vi "Test MultiValue INSERT.vi"(9 "file (use dialog)":path, 10 "Method":T1(ring), 11 "Numeric":i32=1000000) -> (2 "Rows/sec":dbl format="%#_3p", 3 "Time per row":dbl format="%#_3p")   [LabVIEW 2019]
uses:
  <vilib>/JDP Science/PostgreSQL Library/Connection/Execute Command (No results).vi
  <vilib>/JDP Science/PostgreSQL Library/Connection/Execute (no results).vi
  <vilib>/JDP Science/PostgreSQL Library/Connection/Execute (Return first result with rows).vi
  <vilib>/JDP Science/PostgreSQL Library/Connection/Execute Command (Result).vi
  <vilib>/JDP Science/PostgreSQL Library/Result/Clear.vi
  <vilib>/JDP Science/PostgreSQL Library/Connection/Execute Single Statement (String Parameters).vi
  <userlib>/_OpenG.lib/string/string.llb/Trim Whitespace (String)__ogtk.vi
  <vilib>/JDP Science/PostgreSQL Library/Connection/PQ Connection.lvclass
panel:
  out "concatenated string":string
  in  "Connection Strings to access PostgreSQL":string="host=localhost port=5432 dbname = mydb "
  out "error out":errorcluster
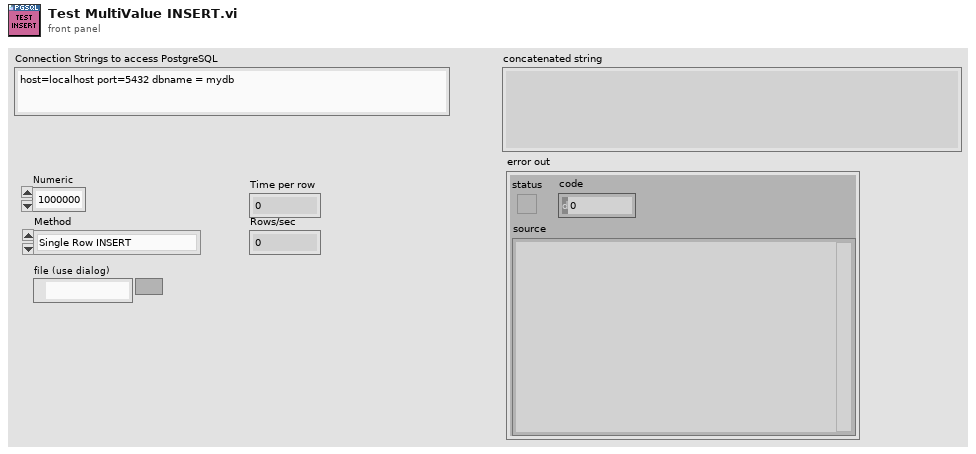
[diagram p1: front panel]
types:
  T1 = enum16{"Single Row INSERT", "Multi Row INSERT", "COPY", "COPY file"}
  T2 = typedef "PQ Result.lvclass/Parameter Type.ctl" = enum16{"Text", "ByteA", "Integer", "SGL", "DBL", "Timestamp", "Enum", "Boolean", "Array", "NULL", "Unsupported"}
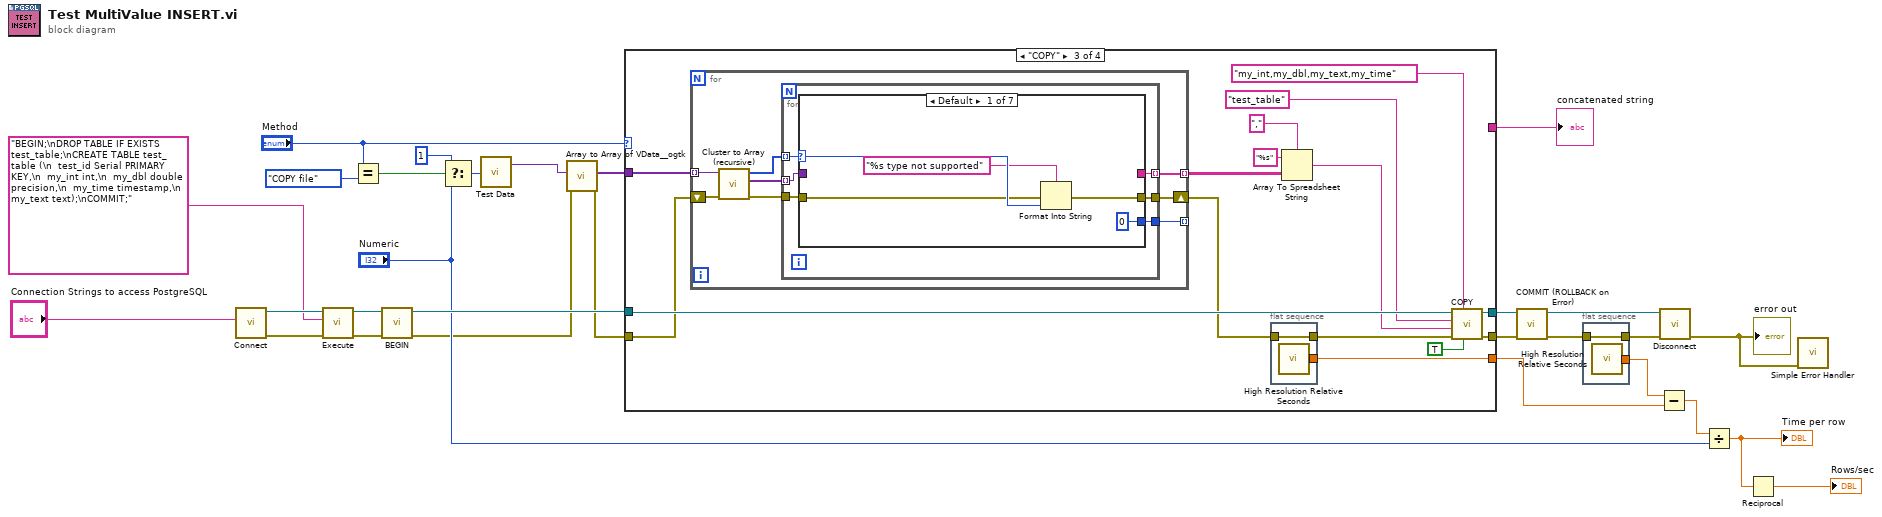
[diagram p0: block diagram]
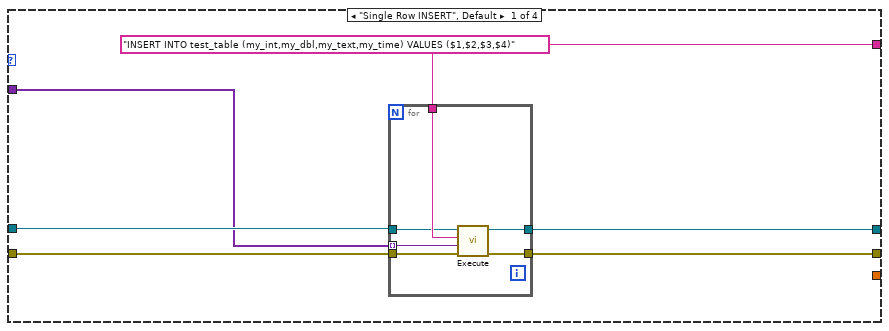
[diagram p2: hidden frame]
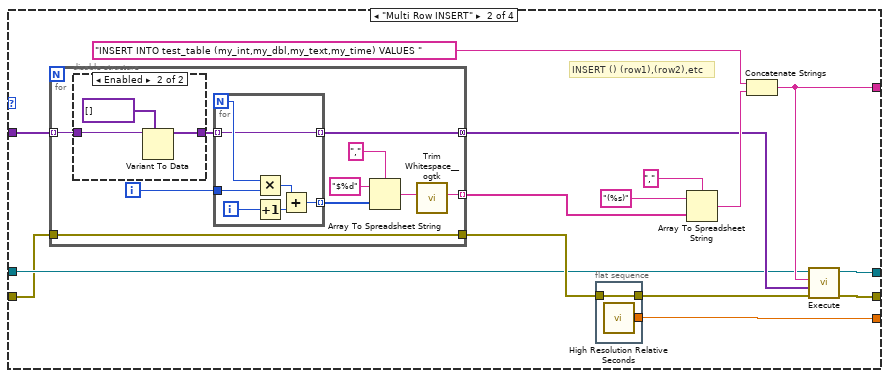
[diagram p3: hidden frame]
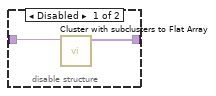
[diagram p4: hidden frame]
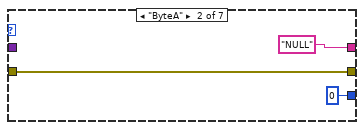
[diagram p5: hidden frame]
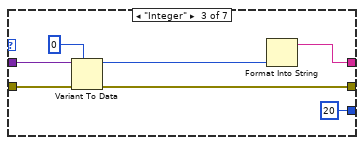
[diagram p6: hidden frame]
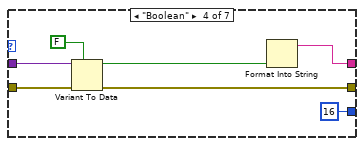
[diagram p7: hidden frame]
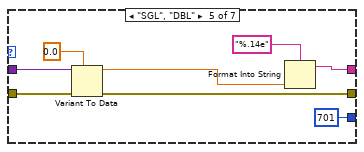
[diagram p8: hidden frame]
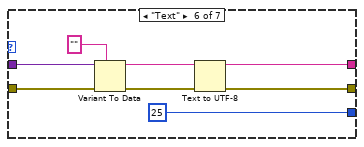
[diagram p9: hidden frame]
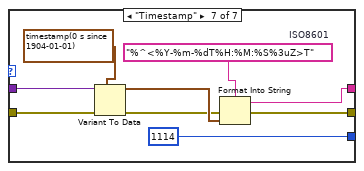
[diagram p10: hidden frame]
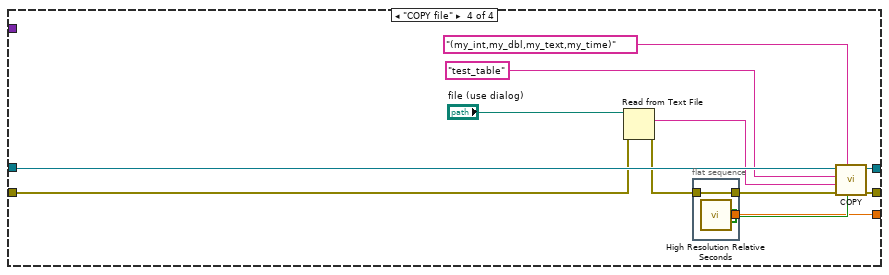
[diagram p11: hidden frame]
diagram:
  n1 = call <vilib>:"Connect.vi"("Connection Strings"="Connection Strings to access PostgreSQL") -> ("error out"=w25:errorcluster, "PQ Connection"=w27:refnum<class "PQ Connection.lvclass">)  [unwired: 9 in]
  n2 = call-poly <vilib>:"Execute.vi"("error in (no error)"=w25, "SQL"="BEGIN;\nDROP TABLE IF EXISTS test_table;\nCREATE TABLE test_table (\n  test_id Serial PRIMARY KEY,\n  my_int int,\n  my_dbl double precision,\n  my_time timestamp,\n  my_text text);\nCOMMIT;", "PQ Connection in"=w27) -> ("error out"=w13:errorcluster, "PQ Connection out"=w26:refnum<class "PQ Connection.lvclass">)  [unwired: 7 in]
  n3 = Equal?(x="Method", y=T1."COPY file") -> (x = y?=w9:bool)
  n4 = call <vilib>:"BEGIN.vi"("error in (no error)"=w13, "PQ Connection in"=w26) -> ("error out"=w2:errorcluster, "PQ Connection out"=w6:refnum<class "PQ Connection.lvclass">)  [unwired: 8 in]
  n5 = Select(t=1, s=w9, f="Numeric") -> (s? t:f=w8:i32)
  n6 = call "Test Data.vi"("Size"=w8) -> ("Data"=w14:variant)  [unwired: 1 out]
  n7 = call <userlib>:"Array to Array of VData__ogtk.vi"("error in (no error)"=w2, "MultiD Array"=w14) -> ("error out"=w1:errorcluster, "1D Array of Variants"=w3:variant[])  [unwired: 8 in]
  n8 = case shown="\"COPY\"" "Method" {
    tunnel: w3 -> [w31 w44 w83 _]
    tunnel: w6 -> [w34 w45 w95 w170]
    tunnel: [w32 w52 w93 w168] -> w17
    tunnel: [w33 w51 w94 w169] -> w16
    tunnel: w1 -> [w35 w43 w82 w160]
    tunnel: [w30 w50 _ _] -> w15
    tunnel: [_ w46 w84 w161] -> w7
    frame "Single Row INSERT", Default {
      w30 = "INSERT INTO test_table (my_int,my_dbl,my_text,my_time) VALUES ($1,$2,$3,$4)" ("command")
      n9 = for {
        tunnel: w30 -> [w40]
        tunnel: w31 -> [w36] mode=indexing
        tunnel: w34 -> [w39]
        tunnel: [w41] -> w32
        tunnel: w35 -> [w38]
        tunnel: [w37] -> w33
        n10 = call-poly <vilib>:"Execute.vi"("error in (no error)"=w38, "Parameters"=w36, "SQL"=w40, "PQ Connection in"=w39) -> ("error out"=w37:errorcluster, "PQ Connection out"=w41:refnum<class "PQ Connection.lvclass">)  [unwired: 6 in]
      }
    }
    frame "Multi Row INSERT" {
      # "INSERT () (row1),(row2),etc"
      n11 = for {
        tunnel: w44 -> [w68] mode=indexing
        tunnel: [w60] -> w42 mode=indexing
        tunnel: [w61] -> w49 mode=concatenating
        tunnel: w43 -> [w59]
        tunnel: [w59] -> w48
        i -> [w66]
        n12 = disable-structure shown="Enabled" {
          disable-tunnel: w68 -> [w70 w72]
          disable-tunnel: [w69 w71] -> w67
          frame Disabled {
            n13 = call <vilib>:"Cluster with subclusters to Flat Array.vi"("Variant"=w70) -> ("Array of items"=w69:variant[])  [unwired: 8 in, 2 out]
          }
          frame Enabled {
            n14 = Variant To Data(type=variant[] [], Variant=w72) -> (data=w71:variant[])  [unwired: 1 in, 1 out]
          }
        }
        n15 = for {
          N -> [w79]
          tunnel: w67 -> [w75] mode=indexing
          tunnel: w66 -> [w78]
          tunnel: [w76] -> w65 mode=indexing
          tunnel: [w75] -> w61 mode=indexing
          i -> [w80]
          n16 = Multiply(x=w79, y=w78) -> (x*y=w77:i32)
          n17 = Increment(x=w80) -> (x+1=w74:i32)
          n18 = Add(x=w77, y=w74) -> (x+y=w76:i32)
        }
        n19 = Array To Spreadsheet String(delimiter (Tab)=",", array=w65, 3:"$%d" ("format string")) -> (spreadsheet string=w62:string)
        n20 = call-poly <userlib>:"Trim Whitespace__ogtk.vi"("String in"=w62) -> ("String out"=w60:string)  [unwired: 6 in]
      }
      n21 = flat-sequence {
        tunnel: w48 -> [w58]
        tunnel: [w58] -> w47
        tunnel: [w57] -> w46
        frame #0 {
          n22 = call <vilib>:"High Resolution Relative Seconds.vi"() -> ("relative seconds"=w57:dbl)
        }
      }
      n23 = Array To Spreadsheet String(delimiter (Tab)=",", array=w42, 3:"(%s)" ("format string")) -> (spreadsheet string=w53:string)
      n24 = Concatenate Strings("INSERT INTO test_table (my_int,my_dbl,my_text,my_time) VALUES " ("command"), w53) -> (w50:string)
      n25 = call-poly <vilib>:"Execute.vi"("error in (no error)"=w47, "Parameters"=w49, "SQL"=w50, "PQ Connection in"=w45) -> ("error out"=w51:errorcluster, "PQ Connection out"=w52:refnum<class "PQ Connection.lvclass">)  [unwired: 6 in]
    }
    frame "COPY" {
      n26 = for {
        tunnel: [w105] -> w91 mode=indexing
        shift-right: [w104] -> w81
        shift-left: w82 -> [w102]
        tunnel: [w103] -> _ mode=indexing
        tunnel: w83 -> [w101] mode=indexing
        n27 = call <vilib>:"Cluster to Array (recursive).vi"("error in (no error)"=w102, "Variant"=w101) -> ("error out"=w98:errorcluster, "Elements"=w100:variant[], "Types"=w99:T2[])  [unwired: 6 in, 1 out]
        n28 = for {
          tunnel: [w111] -> w105 mode=indexing
          tunnel: [w110] -> w104
          tunnel: [w109] -> w103
          tunnel: w100 -> [w107] mode=indexing
          tunnel: w99 -> [w108] mode=indexing
          tunnel: w98 -> [w106]
          n29 = case shown="Default" w108 {
            selector: w108 -> [w116 _ _ _ _ _ _]
            tunnel: w107 -> [_ _ w126 w133 w141 w149 w158]
            tunnel: [_ "NULL" w123 w131 w138 w144 w150] -> w111
            tunnel: w106 -> [w114 w118 w122 w130 w136 w147 w157]
            tunnel: [w113 w118 w121 w129 w135 w142 w151] -> w110
            tunnel: [0 0 20 16 701 25 1114] -> w109
            frame Default {
              n30 = Format Into String(format string="%s type not supported", error in=w114, w116) -> (error out=w113:errorcluster)  [unwired: 1 in, 1 out]
            }
            frame "ByteA" {
            }
            frame "Integer" {
              n31 = Variant To Data(error in=w122, type=i64 0, Variant=w126) -> (data=w124:i64, error out=w121:errorcluster)
              n32 = Format Into String(w124) -> (resulting string=w123:string)  [unwired: 3 in, 1 out]
            }
            frame "Boolean" {
              n33 = Variant To Data(error in=w130, type=FALSE, Variant=w133) -> (data=w132:bool, error out=w129:errorcluster)
              n34 = Format Into String(w132) -> (resulting string=w131:string)  [unwired: 3 in, 1 out]
            }
            frame "SGL", "DBL" {
              n35 = Variant To Data(error in=w136, type=0.0, Variant=w141) -> (data=w139:dbl, error out=w135:errorcluster)
              n36 = Format Into String(format string="%.14e", w139) -> (resulting string=w138:string)  [unwired: 2 in, 1 out]
            }
            frame "Text" {
              n37 = Variant To Data(error in=w147, type="", Variant=w149) -> (data=w145:string, error out=w143:errorcluster)
              n38 = Text to UTF-8(8:w143, 11:w145) -> (0:w142:errorcluster, 3:w144:string)  [unwired: 1 in]
            }
            frame "Timestamp" {
              w154 = "%^<%Y-%m-%dT%H:%M:%S%3uZ>T"  # ISO8601
              n39 = Variant To Data(error in=w157, type=timestamp(0 s since 1904-01-01), Variant=w158) -> (data=w153:timestamp, error out=w152:errorcluster)
              n40 = Format Into String(format string=w154, error in=w152, w153) -> (resulting string=w150:string, error out=w151:errorcluster)  [unwired: 1 in]
            }
          }
        }
      }
      n41 = flat-sequence {
        tunnel: w81 -> [w97]
        tunnel: [w97] -> w85
        tunnel: [w96] -> w84
        frame #0 {
          n42 = call <vilib>:"High Resolution Relative Seconds.vi"() -> ("relative seconds"=w96:dbl)
        }
      }
      n43 = Array To Spreadsheet String(delimiter (Tab)=",", array=w91, 3:"%s" ("format string")) -> (spreadsheet string=w86:string)
      n44 = call <vilib>:"COPY.vi"("CSV?"=TRUE, "column name(s) (empty=ALL)"="my_int,my_dbl,my_text,my_time" ("command"), "error in (no error)"=w85, "buffer"=w86, "table name"="test_table" ("command"), "PQ Connection in"=w95) -> ("error out"=w94:errorcluster, "PQ Connection out"=w93:refnum<class "PQ Connection.lvclass">)  [unwired: 4 in]
    }
    frame "COPY file" {
      n45 = Read from Text File(file (use dialog)="file (use dialog)", error in=w160) -> (text=w164:string, error out=w159:errorcluster)  [unwired: 2 in, 2 out]
      n46 = flat-sequence {
        tunnel: w159 -> [w172]
        tunnel: [w172] -> w162
        tunnel: [w171] -> w161
        frame #0 {
          n47 = call <vilib>:"High Resolution Relative Seconds.vi"() -> ("relative seconds"=w171:dbl)
        }
      }
      n48 = call <vilib>:"COPY.vi"("CSV?"=TRUE, "column name(s) (empty=ALL)"="(my_int,my_dbl,my_text,my_time)" ("command"), "error in (no error)"=w162, "buffer"=w164, "table name"="test_table" ("command"), "PQ Connection in"=w170) -> ("error out"=w169:errorcluster, "PQ Connection out"=w168:refnum<class "PQ Connection.lvclass">)  [unwired: 4 in]
    }
  }
  "concatenated string" <- w15
  n49 = call <vilib>:"COMMIT (ROLLBACK on Error).vi"("error in (no error)"=w16, "PQ Connection in"=w17) -> ("error out"=w22:errorcluster, "PQ Connection out"=w23:refnum<class "PQ Connection.lvclass">)  [unwired: 8 in]
  n50 = flat-sequence {
    tunnel: w22 -> [w174]
    tunnel: [w174] -> w21
    tunnel: [w173] -> w20
    frame #0 {
      n51 = call <vilib>:"High Resolution Relative Seconds.vi"() -> ("relative seconds"=w173:dbl)
    }
  }
  n52 = Subtract(x=w20, y=w7) -> (x-y=w12:dbl)
  n53 = call <vilib>:"Disconnect.vi"("error in (no error)"=w21, "PQ Connection in"=w23) -> ("error out"=w28:errorcluster)  [unwired: 9 in]
  "error out" <- w28
  n54 = Divide(x=w12, y="Numeric") -> (x/y=w19:dbl)
  "Time per row" <- w19
  n55 = Reciprocal(x=w19) -> (1/x=→"Rows/sec":dbl)
  n56 = call <vilib>:"Simple Error Handler.vi"("error in (no error)"=w28) -> ()  [unwired: 4 in, 5 out]
